vi "B軸回home_function.vi"(7 "B¶b Home_action":T1, 8 "error in (no error)":errorcluster) -> (0 "error out":errorcluster)   [LabVIEW 2014]
uses:
  global/Global.vi
panel:
  out "state":u8
  # "B軸為塑膠蓋的夾爪"
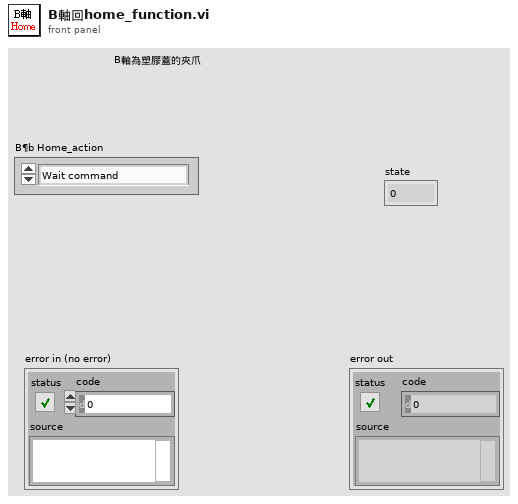
[diagram p1: front panel]
types:
  T1 = typedef "B¶b home_action.ctl" = enum16{"Wait command", "Config phi motor", "Start phi homing", "確認 phi homing done", "error"}
  T2 = typedef "home function.ctl" = enum16{"Wait command", "Config X home mode_7", "Start X homing_7", "確認 X homing_7 done", "Config Y home mode_7", "Start Y homing_7", "確認 Y homing_7 done", "Config Z home mode_7", "Start Z homing_7", "確認 Z homing_7 done", "Config phi motor", "Start phi homing", "確認 phi homing done", "finish", "error"}
  T3 = typedef "軸參數記錄.ctl" = cluster{"X軸取料位":dbl, "X¶bCCD¦ì":dbl, "X軸影像異常排料位":dbl, "X軸迴轉缸位":dbl, "裝完料區已可安全取料位":dbl, "A軸取料角":dbl, "A¶bCCD¨¤":dbl, "B軸取料角":dbl, "B¶bCCD¨¤":dbl, "軸控參數PATH":path, "CCD左連續失敗報警次數":u8, "CCD右連續失敗報警次數":u8, "連續組裝失敗報警次數":u8, "ABVL/VH":i32, "XVL/VH":i32, "AB加速度":i32, "X加速度":i32, "home-XVL/VH":i32, "home-ABVL/VH":i32}
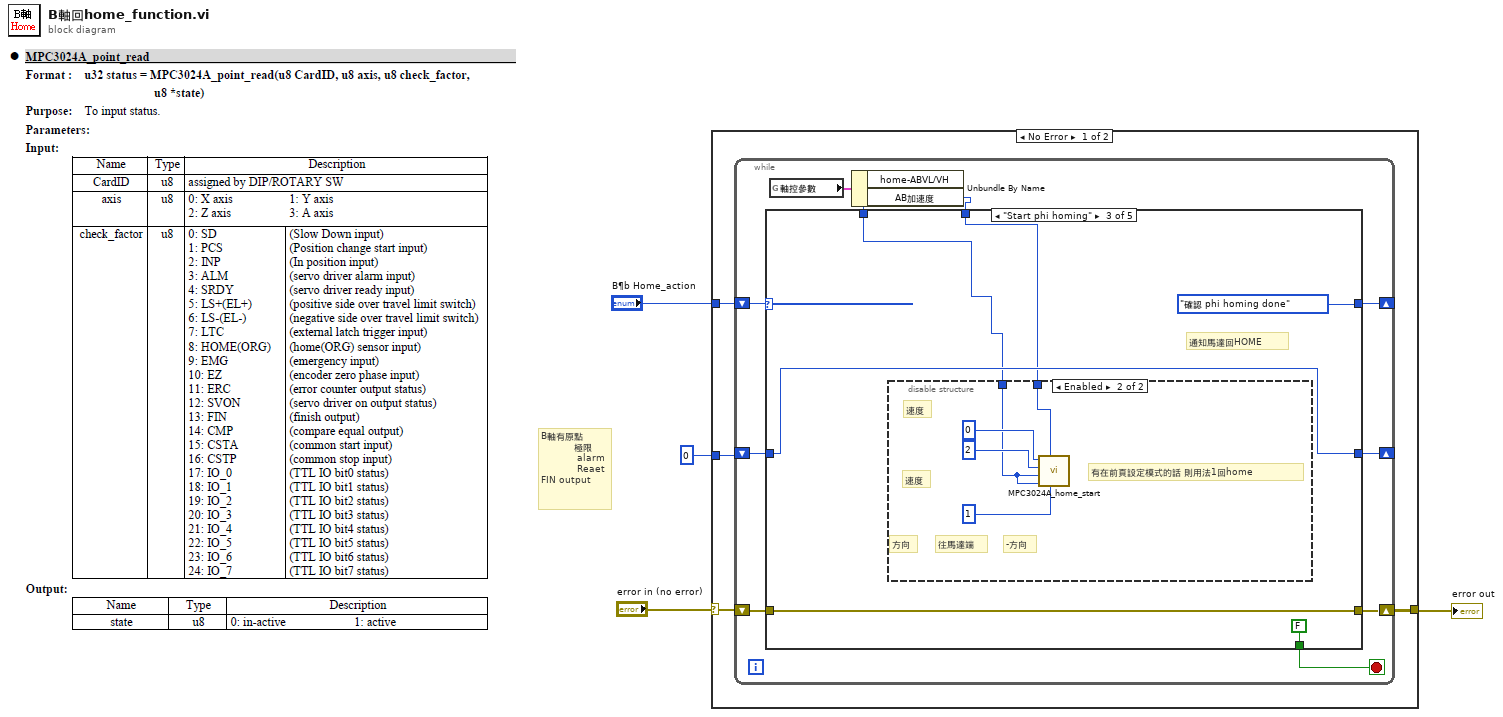
[diagram p0: block diagram]
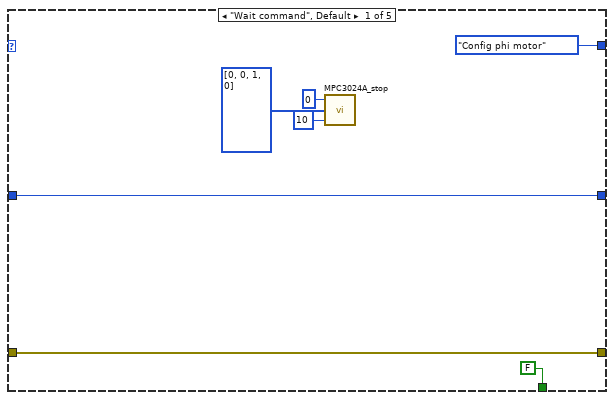
[diagram p2: hidden frame]
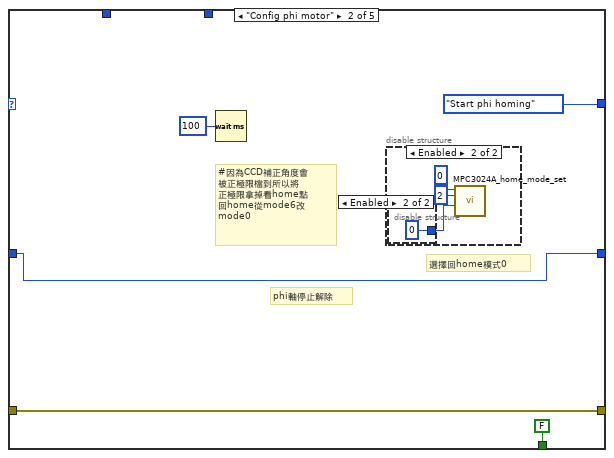
[diagram p3: hidden frame]
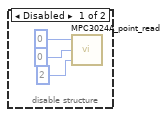
[diagram p4: hidden frame]
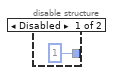
[diagram p5: hidden frame]
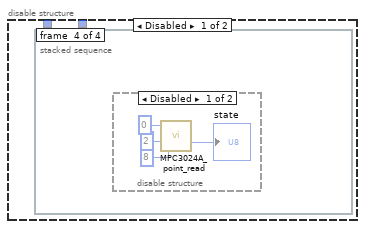
[diagram p6: hidden frame]
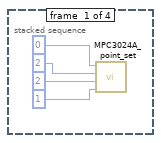
[diagram p7: hidden frame]
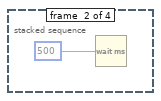
[diagram p8: hidden frame]
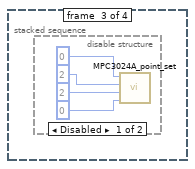
[diagram p9: hidden frame]
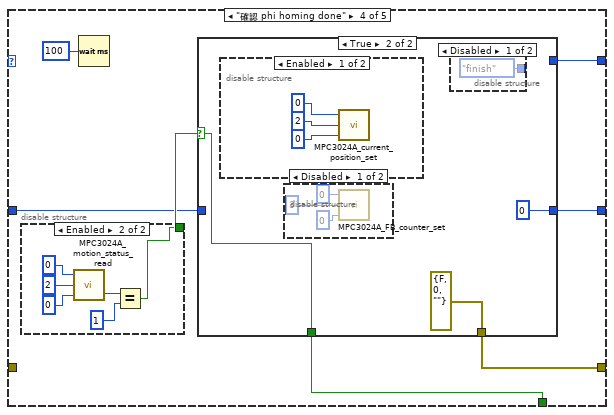
[diagram p12: hidden frame]
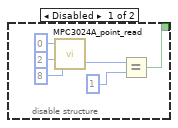
[diagram p13: hidden frame]
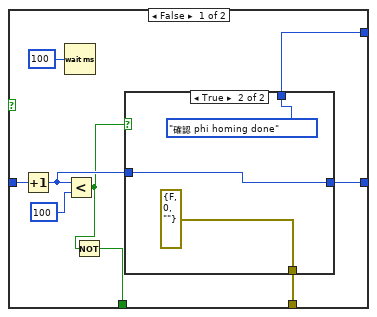
[diagram p14: hidden frame]
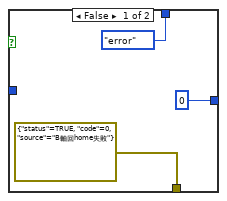
[diagram p15: hidden frame]
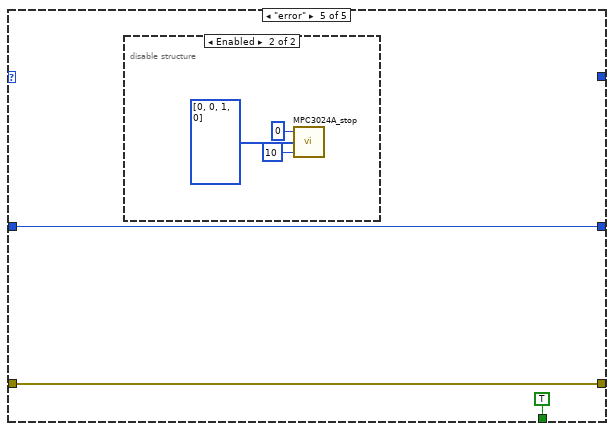
[diagram p19: hidden frame]
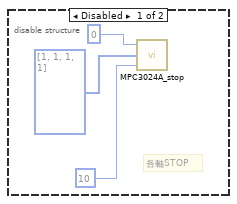
[diagram p20: hidden frame]
diagram:
  # "B軸有原點\n           極限\n            alarm\n            Reaet\nFIN output"
  n1 = case shown="No Error" "error in (no error)" {
    selector: "error in (no error)" -> [w7 w116]
    tunnel: [w6 w116] -> w3
    tunnel: "B¶b Home_action" -> [w8 _]
    tunnel: 0 -> [w5 _]
    frame No Error {
      n2 = while {
        shift-right: [w17] -> _
        shift-left: w8 -> [w18]
        shift-right: [w14] -> w6
        shift-left: w7 -> [w15]
        shift-right: [w12] -> _
        shift-left: w5 -> [w13]
        stop <- w16 stop-if-true
        n3 = global read "Global.vi" "軸控參數"() -> (w11:T3)
        n4 = Unbundle By Name(w11) -> ("home-ABVL/VH"=w10:i32, "AB加速度"=w9:i32)
        n5 = case shown="\"Start phi homing\"" w18 {
          tunnel: [B¶b_home_action."Config phi motor" ("B¶b Home_action") B¶b_home_action."Start phi homing" ("B¶b Home_action") B¶b_home_action."確認 phi homing done" ("B¶b Home_action") w63 _] -> w17
          tunnel: [FALSE FALSE FALSE w64 TRUE] -> w16
          tunnel: w15 -> [w24 w28 w44 _ w108]
          tunnel: [w24 w28 w44 w65 w108] -> w14
          tunnel: w13 -> [w23 w27 w42 w67 w109]
          tunnel: [w23 w27 w42 w66 w109] -> w12
          tunnel: w10 -> [_ _ w40 _ _]
          tunnel: w9 -> [_ _ w39 _ _]
          frame "Wait command", Default {
            n6 = call "MPC3024A_stop.vi"("Tdec_ms"=u32 10, "axis[4]"=u8[] [0, 0, 1, 0], "CardID"=u8 0) -> ()  [unwired: 1 out]
          }
          frame "Config phi motor" {
            # "#因為CCD補正角度會\n被正極限檔到所以將\n正極限拿掉看home點\n回home從mode6改\nmode0"
            # "選擇回home模式0"
            # "phi軸停止解除"
            n7 = Wait (ms)(milliseconds to wait=u32 100) -> ()  [unwired: 1 out]
            n8 = disable-structure shown="Enabled" {
              frame Disabled {
                n9 = call "MPC3024A_point_read.vi"("check_factor"=u8 2, "axis"=u8 0, "CardID"=u8 0) -> ()  [unwired: 2 out]
              }
              frame Enabled {
                n10 = disable-structure shown="Enabled" {
                  disable-tunnel: [u8 1 ("mode") u8 0 ("mode")] -> w34
                  frame Disabled {
                  }
                  frame Enabled {
                  }
                }
                n11 = call "MPC3024A_home_mode_set.vi"("mode"=w34, "axis"=u8 2, "CardID"=u8 0) -> ()  [unwired: 1 in, 1 out]
              }
            }
          }
          frame "Start phi homing" {
            # "通知馬達回HOME"
            n12 = disable-structure shown="Enabled" {
              disable-tunnel: w40 -> [_ w59]
              disable-tunnel: w39 -> [_ w58]
              frame Disabled {
                n13 = stacked-sequence {
                  frame #0 {
                    n14 = call "MPC3024A_point_set.vi"("on_off"=u8 1, "check_factor"=u8 2, "axis"=u8 2, "CardID"=u8 0) -> ()  [unwired: 1 out]
                  }
                  frame #1 {
                    n15 = Wait (ms)(milliseconds to wait=u32 500) -> ()  [unwired: 1 out]
                  }
                  frame #2 {
                    n16 = disable-structure shown="Disabled" {
                      frame Disabled {
                        n17 = call "MPC3024A_point_set.vi"("on_off"=u8 0, "check_factor"=u8 2, "axis"=u8 2, "CardID"=u8 0) -> ()  [unwired: 1 out]
                      }
                      frame Enabled {
                      }
                    }
                  }
                  frame #3 {
                    n18 = disable-structure shown="Disabled" {
                      frame Disabled {
                        n19 = call "MPC3024A_point_read.vi"("check_factor"=u8 8, "axis"=u8 2, "CardID"=u8 0) -> ("state"=→"state":u8)  [unwired: 1 out]
                      }
                      frame Enabled {
                      }
                    }
                  }
                }
              }
              frame Enabled {
                # "-方向"
                # "往馬達端"
                # "有在前頁設定模式的話 則用法1回home"
                # "速度"
                # "速度"
                # "方向"
                n20 = call "MPC3024A_home_start.vi"("direction"=u8 1, "Tacc_ms"=w58, "VH"=w59, "VL"=w59, "axis"=u8 2, "CardID"=u8 0) -> ()  [unwired: 1 out]
              }
            }
          }
          frame "確認 phi homing done" {
            n21 = disable-structure shown="Enabled" {
              disable-tunnel: [w71 w76] -> w69
              frame Disabled {
                n22 = call "MPC3024A_point_read.vi"("check_factor"=u8 8, "axis"=u8 2, "CardID"=u8 0) -> ("state"=w75:u8)  [unwired: 1 out]
                n23 = Equal?(x=w75, y=u8 1) -> (x = y?=w71:bool)
              }
              frame Enabled {
                n24 = call "MPC3024A_motion_status_read.vi"("check_factor"=u8 0, "axis"=u8 2, "CardID"=u8 0) -> ("ret_fig"=w81:u8)  [unwired: 1 out]
                n25 = Equal?(x=w81, y=u8 1) -> (x = y?=w76:bool)
              }
            }
            n26 = Wait (ms)(milliseconds to wait=u32 100) -> ()  [unwired: 1 out]
            n27 = case shown="True" w69 {
              selector: w69 -> [_ w97]
              tunnel: w67 -> [w90 _]
              tunnel: [w88 0] -> w66
              tunnel: [w86 errorcluster {"status"=FALSE, "code"=0, "source"=""} ("error in (no error)")] -> w65
              tunnel: [w83 w97] -> w64
              tunnel: [w82 _] -> w63
              frame False {
                n28 = Increment(x=w90) -> (x+1=w87:i32)
                n29 = Wait (ms)(milliseconds to wait=u32 100) -> ()  [unwired: 1 out]
                n30 = Less?(x=w87, y=100) -> (x < y?=w84:bool)
                n31 = Not(x=w84) -> (.not. x?=w83:bool)
                n32 = case shown="True" w84 {
                  tunnel: [0 w96] -> w88
                  tunnel: w87 -> [_ w96]
                  tunnel: [errorcluster {"status"=TRUE, "code"=0, "source"="B軸回home失敗"} ("error in (no error)") errorcluster {"status"=FALSE, "code"=0, "source"=""} ("error in (no error)")] -> w86
                  tunnel: [B¶b_home_action."error" ("B¶b Home_action") B¶b_home_action."確認 phi homing done" ("B¶b Home_action")] -> w82
                  frame False {
                  }
                  frame True {
                  }
                }
              }
              frame True {
                n33 = disable-structure shown="Enabled" {
                  frame Enabled {
                    n34 = call "MPC3024A_current_position_set.vi"("current_posi"=0, "axis"=u8 2, "CardID"=u8 0) -> ()  [unwired: 1 out]
                  }
                  frame Disabled {
                  }
                }
                n35 = disable-structure shown="Disabled" {
                  frame Disabled {
                    n36 = call "MPC3024A_FB_counter_set.vi"("value"=0, "axis"=u8 3, "CardID"=u8 0) -> ()  [unwired: 1 out]
                  }
                  frame Enabled {
                  }
                }
                n37 = disable-structure shown="Disabled" {
                  disable-tunnel: [home_function."finish" ("Home function") _] -> _
                  frame Disabled {
                  }
                  frame Enabled {
                  }
                }
              }
            }
          }
          frame "error" {
            n38 = disable-structure shown="Enabled" {
              frame Disabled {
                # "各軸STOP"
                n39 = call "MPC3024A_stop.vi"("Tdec_ms"=u32 10, "axis[4]"=u8[] [1, 1, 1, 1], "CardID"=u8 0) -> ()  [unwired: 1 out]
              }
              frame Enabled {
                n40 = call "MPC3024A_stop.vi"("Tdec_ms"=u32 10, "axis[4]"=u8[] [0, 0, 1, 0], "CardID"=u8 0) -> ()  [unwired: 1 out]
              }
            }
          }
        }
      }
    }
    frame Error {
    }
  }
  "error out" <- w3
